vi "Convert UIMsg Event.vi"(11 "UIMsg Event":i32) -> (3 "UIMsg":T1, 5 "String Value":string)   [LabVIEW 2020, in "HTS.lvlib"]
uses:
  HTS.lvlib
  Data Types/UIMsg.ctl
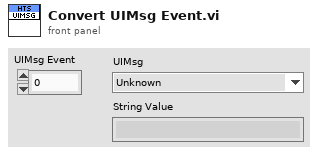
[diagram p1: front panel]
types:
  T1 = typedef "HTS.lvlib/UIMsg.ctl" = enum16{"Unknown", "BreakOnUserRequest", "BreakOnBreakpoint", "BreakOnRunTimeError", "Trace", "TerminatingExecution", "AbortingExecution", "KillingExecutionThreads", "EndExecution", "ShutDownComplete", "StartExecution", "ProgressPercent", "ProgressText", "StartInteractiveExecution", "EndInteractiveExecution", "TerminatingInteractiveExecution", "TerminationCancelled", "ResumeFromBreak", "StartFileExecution", "EndFileExecution", "ShutDownCancelled", "LocalizationSettingChanged", "OpenWindows", "TileWindows", "CascadeWindows", "ReportChanged", "CloseWindows", "RefreshWindows", "ClientFileChanged", "DisplayReport", "ModelState_Initializing", "ModelState_Waiting", "ModelState_Identified", "ModelState_BeginTesting", "ModelState_TestingComplete", "ModelState_PostProcessingComplete", "ModelState_EnabledStateSet", "ReportLocationChanged", "GotoLocation", "PushUndoItem", "OutputMessages", "TypePaletteFileListChanged", "NonTerminatingThreadsArePreventingTermination", "ModelState_PostProcessing", "ReportCollectionChanged", "RuntimeError"}
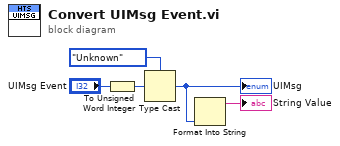
[diagram p0: block diagram]
diagram:
  n1 = To Unsigned Word Integer(number="UIMsg Event") -> (unsigned 16bit integer=w1:u16)
  n2 = Type Cast(type=UIMsg."Unknown" ("UIMsg"), x=w1) -> (*(type *) &x=w3:T1)
  "UIMsg" <- w3
  n3 = Format Into String(w3) -> (resulting string=→"String Value":string)  [unwired: 3 in, 1 out]
